vi "get_UIM_MCFG.vi"(8 "error in (no error)":errorcluster caption="错误输入（无错误）", 11 "StepMotor输入":refnum<class "StepMotor.lvclass">) -> (0 "error out":errorcluster caption="错误输出", 2 "MCFG输入":T1, 3 "StepMotor输出":refnum<class "StepMotor.lvclass">)   [LabVIEW 2016, in "MotionControl.lvlib" / "StepMotor.lvclass"]
uses:
  <userlib>/MotionControl/StepMotor/StepMotor.lvclass
  <userlib>/MotionControl/StepMotor/StepMotor.lvclass/StepMotor.ctl
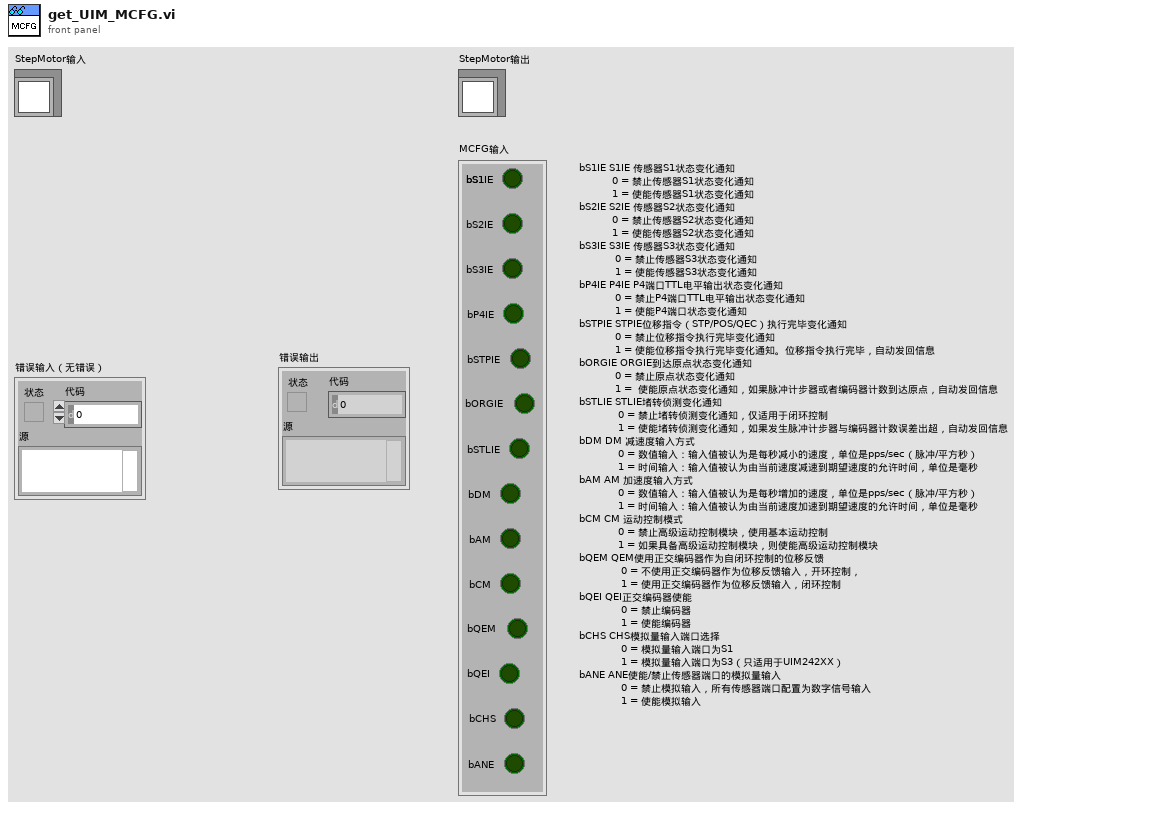
[diagram p1: front panel]
types:
  T1 = cluster{"bS1IE":bool, "bS2IE":bool, "bS3IE":bool, "bP4IE":bool, "bSTPIE":bool, "bORGIE":bool, "bSTLIE":bool, "bDM":bool, "bAM":bool, "bCM":bool, "bQEM":bool, "bQEI":bool, "bCHS":bool, "bANE":bool}
  T2 = typedef "MotionControl.lvlib/StepMotor.lvclass/UIM_MCFG.ctl" = cluster{"bS1IE":bool, "bS2IE":bool, "bS3IE":bool, "bP4IE":bool, "bSTPIE":bool, "bORGIE":bool, "bSTLIE":bool, "bDM":bool, "bAM":bool, "bCM":bool, "bQEM":bool, "bQEI":bool, "bCHS":bool, "bANE":bool}
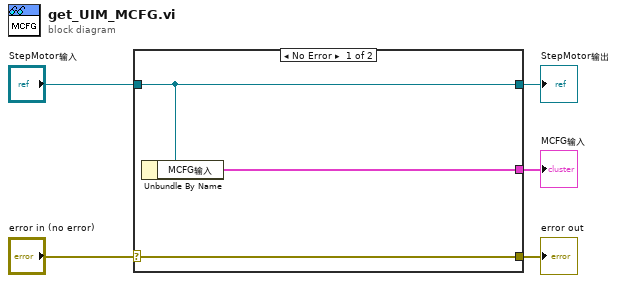
[diagram p0: block diagram]
diagram:
  n1 = case shown="No Error" "error in (no error)" {
    selector: "error in (no error)" -> [w8 w9]
    tunnel: [w8 w9] -> w4
    tunnel: [w7 w10] -> w2
    tunnel: "StepMotor输入" -> [w7 w10]
    tunnel: [w6 _] -> w1
    frame No Error {
      n2 = Unbundle By Name(w7) -> ("MCFG输入"=w6:T2)
    }
    frame Error {
    }
  }
  "error out" <- w4
  "StepMotor输出" <- w2
  "MCFG输入" <- w1
